vi "Test Basic Function 3.vi"() -> ()   [LabVIEW 2014]
uses:
  <vilib>/Aledyne-TSXperts/Arduino Compatible Compiler for LabVIEW/addons/Arduino Math/Arduino Math.lvlib
panel:
  out "fmod(x,y)":sgl
  out "modf(x,frac part)":sgl
  out "cbrt(x)":sgl
  out "hypot(x,y)":sgl
  out "result":sgl
  out "sqrt(x)":sgl
  out "x^2":sgl
  out "Error Out":errorcluster
  in  "Error In":errorcluster
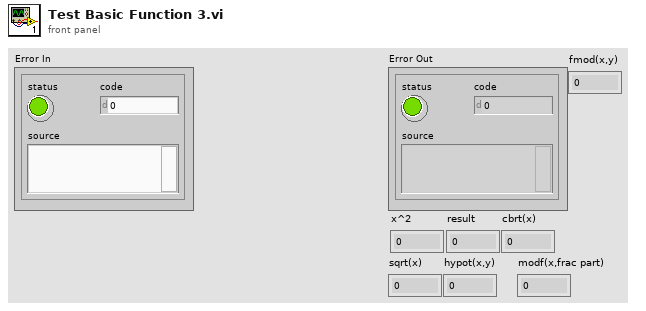
[diagram p1: front panel]
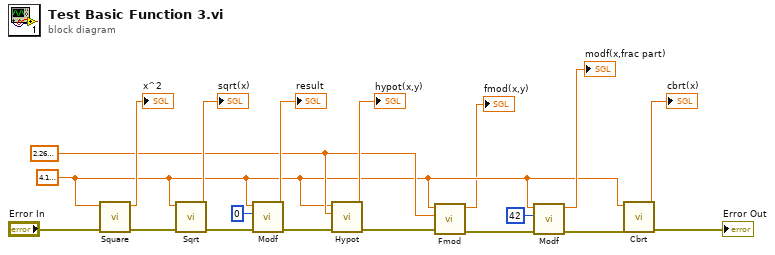
[diagram p0: block diagram]
diagram:
  w3 = sgl 2.27 ("x")
  w2 = sgl 4.2 ("x")
  n1 = call <vilib>:"Square.vi"("Error In"="Error In", "x"=w2) -> ("Error Out"=w17:errorcluster, "x^2"=→"x^2":dbl)  [unwired: 8 in]
  n2 = call <vilib>:"Sqrt.vi"("Error In"=w17, "x"=w2) -> ("Error Out"=w16:errorcluster, "sqrt(x)"=→"sqrt(x)":dbl)  [unwired: 8 in]
  n3 = call <vilib>:"Modf.vi"("Error In"=w16, "y"=u32 0, "x"=w2) -> ("Error Out"=w15:errorcluster, "modf(x,frac part)"=→"result":dbl)  [unwired: 7 in]
  n4 = call <vilib>:"Hypot.vi"("Error In"=w15, "y"=w3, "x"=w2) -> ("Error Out"=w5:errorcluster, "hypot(x,y)"=→"hypot(x,y)":dbl)  [unwired: 7 in]
  n5 = call <vilib>:"Fmod.vi"("Error In"=w5, "y"=w3, "x"=w2) -> ("Error Out"=w4:errorcluster, "fmod(x,y)"=→"fmod(x,y)":dbl)  [unwired: 7 in]
  n6 = call <vilib>:"Modf.vi"("Error In"=w4, "y"=u32 42, "x"=w2) -> ("Error Out"=w8:errorcluster, "modf(x,frac part)"=→"modf(x,frac part)":dbl)  [unwired: 7 in]
  n7 = call <vilib>:"Cbrt.vi"("Error In"=w8, "x"=w2) -> ("Error Out"=→"Error Out":errorcluster, "cbrt(x)"=→"cbrt(x)":dbl)  [unwired: 8 in]
